vi "2.更新信息.vi"(8 "error in":errorcluster, 10 "Message":string, 11 "Module ID":i32=-1) -> (0 "error out":errorcluster, 3 "Module ID out":i32=-1)   [LabVIEW 2020, in "Log.lvlib"]
uses:
  Log.lvlib
  Log.lvlibp
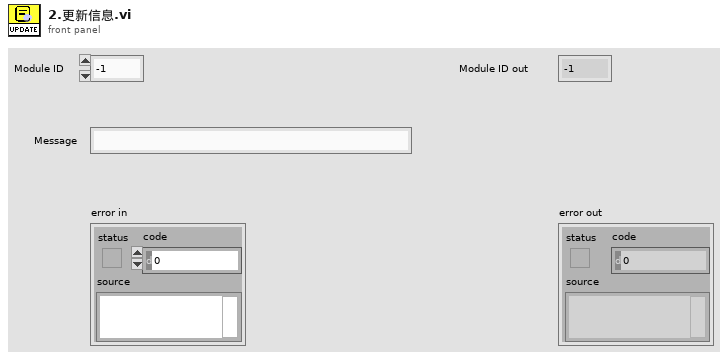
[diagram p1: front panel]
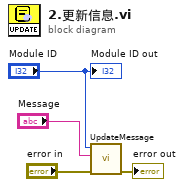
[diagram p0: block diagram]
diagram:
  n1 = call "UpdateMessage.vi"("error in"="error in", "Message"="Message", "Module ID"="Module ID") -> ("error out"=→"error out":errorcluster)  [unwired: 8 in]
  "Module ID out" <- "Module ID"
